vi "Display FB Seq.vi"(10 "ALS AO in":dbl[](array[numeric]), 11 "ALS DO in":bool[](array[boolean])) -> (2 "AO State":cluster{"DO":dbl, "CN":string}[](array[cluster]), 3 "DO State":cluster{"DO":bool, "CN":string}[](array[cluster]))   [LabVIEW 2022 SP3]
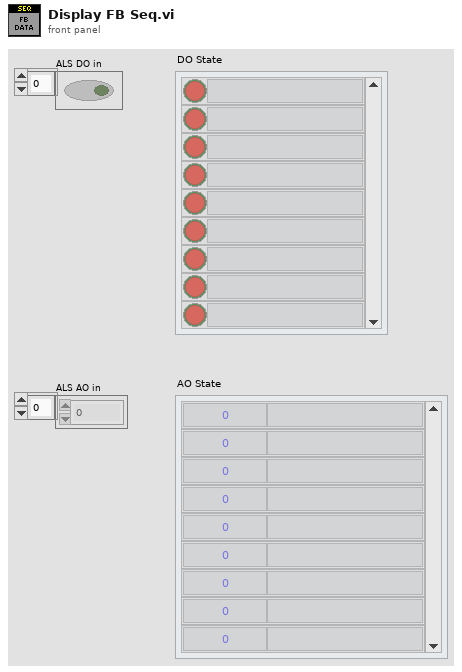
[diagram p1: front panel]
types:
  T1 = cluster{"AO Names":string[], "AI Names":string[], "DI Names":string[], "DO Names":string[], "TC Names":string[], "AO Default":dbl[], "DO Default":bool[], "ACC Names":string[], "SG Names":string[]}
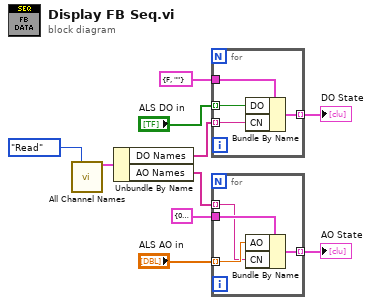
[diagram p0: block diagram]
diagram:
  n1 = call "All Channel Names.vi"("Enum"=enum16{"Read", "Write"}."Read") -> ("Channel names"=w6:T1)  [unwired: 13 in, 1 out]
  n2 = Unbundle By Name(w6) -> ("DO Names"=w7:string[], "AO Names"=w9:string[])
  n3 = for {
    tunnel: "ALS DO in" -> [w13] mode=indexing
    tunnel: cluster{"DO":bool, "CN":string} {"DO"=FALSE, "CN"=""} ("DO") -> [w14]
    tunnel: [w12] -> w8 mode=indexing
    tunnel: w7 -> [w11] mode=indexing
    n4 = Bundle By Name(cluster=w14, "DO"=w13, "CN"=w11) -> (w12:cluster{"DO":bool, "CN":string})
  }
  "DO State" <- w8
  n5 = for {
    tunnel: cluster{"AO":dbl, "CN":string} {"AO"=0.0, "CN"=""} ("DO") -> [w18]
    tunnel: [w17] -> w2 mode=indexing
    tunnel: "ALS AO in" -> [w16] mode=indexing
    tunnel: w9 -> [w15] mode=indexing
    n6 = Bundle By Name(cluster=w18, "AO"=w16, "CN"=w15) -> (w17:cluster{"AO":dbl, "CN":string})
  }
  "AO State" <- w2
